vi "height set.vi"(6 "offset":dbl, 10 "height name":T1, 11 "plus in":bool) -> (3 "Numeric":dbl)   [LabVIEW 2019]
uses:
  ctl/height.ctl
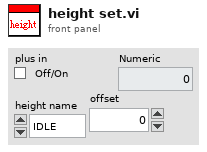
[diagram p1: front panel]
types:
  T1 = typedef "height.ctl" = enum16{"IDLE", "recycle pre-catch", "recycle catch", "recycle zone", "vision height", "box 1", "box 2", "box 3", "box 1 pre", "box 2 pre", "box 3 pre", "reg 1", "reg 2", "reg 1 pre", "reg 2 pre", "put 1", "put 2", "put 3"}
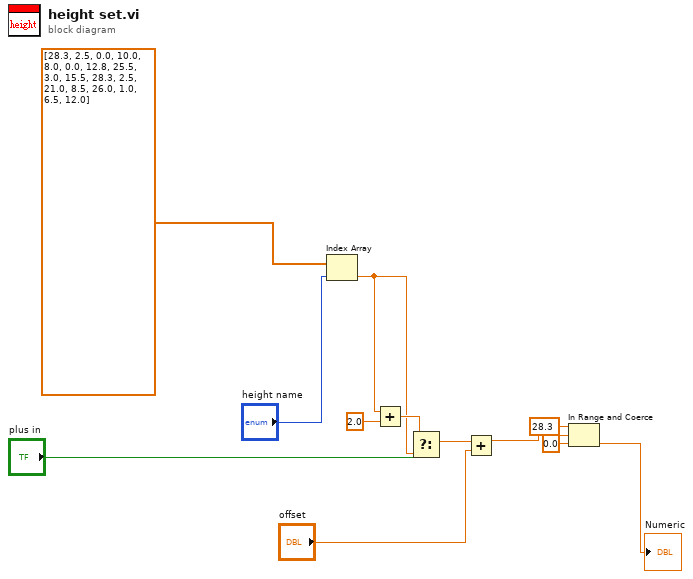
[diagram p0: block diagram]
diagram:
  n1 = Index Array(array=dbl[] [28.3, 2.5, 0.0, 10.0, 8.0, 0.0, 12.8, 25.5, 3.0, 15.5, 28.3, 2.5, 21.0, 8.5, 26.0, 1.0, 6.5, 12.0], index="height name") -> (element=w9:dbl)
  n2 = Add(x=w9, y=2.0) -> (x+y=w11:dbl)
  n3 = Select(t=w11, s="plus in", f=w9) -> (s? t:f=w5:dbl)
  n4 = Add(x=w5, y="offset") -> (x+y=w2:dbl)
  n5 = In Range and Coerce(upper limit=28.3, x=w2, lower limit=0.0) -> (coerced(x)=→"Numeric":dbl)  [unwired: 1 out]
